vi "Self Calibrate.vi"(8 "error in (no error)":errorcluster, 11 "LINX-ADS1256 in":refnum<class "LINX-ADS1256.lvclass">) -> (0 "error out":errorcluster, 3 "LINX-ADS1256 out":refnum<class "LINX-ADS1256.lvclass">)   [LabVIEW 2020, in "LINX-ADS1256.lvclass"]
uses:
  LINX-ADS1256.lvclass
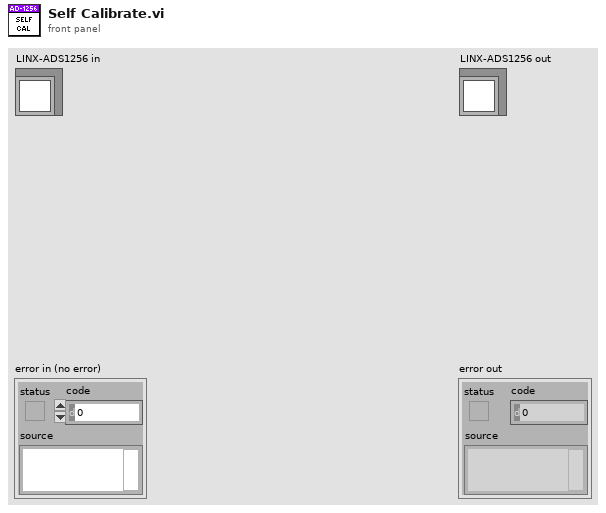
[diagram p1: front panel]
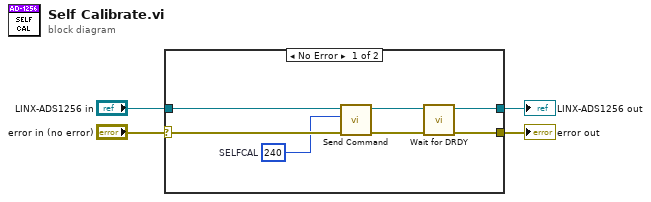
[diagram p0: block diagram]
diagram:
  n1 = case shown="No Error" "error in (no error)" {
    selector: "error in (no error)" -> [w10 w13]
    tunnel: [w7 w13] -> w3
    tunnel: [w6 w12] -> w1
    tunnel: "LINX-ADS1256 in" -> [w11 w12]
    frame No Error {
      w5 = u8 240  # SELFCAL
      n2 = call "Send Command.vi"("error in (no error)"=w10, "Register Address"=w5, "LINX-ADS1256 in"=w11) -> ("error out"=w8:errorcluster, "LINX-ADS1256 out"=w9:refnum<class "LINX-ADS1256.lvclass">)  [unwired: 7 in]
      n3 = call "Wait for DRDY.vi"("error in (no error)"=w8, "LINX-ADS1256 in"=w9) -> ("error out"=w7:errorcluster, "LINX-ADS1256 out"=w6:refnum<class "LINX-ADS1256.lvclass">)  [unwired: 6 in, 2 out]
    }
    frame Error {
    }
  }
  "error out" <- w3
  "LINX-ADS1256 out" <- w1
